vi "QuickSearch Demo.vi"() -> ()   [LabVIEW 2018]
panel:
  in  "Command":string(combo)
  in  "Name Match List":i32(listbox)
  in  "Forward":bool
  in  "Name Match List Ref":refnum<vi>
  in  "Object Name Ref":refnum<vi>
  out "Selected String":string
  out "Shortcuts":string[](array[string])
  in  "vi reference":refnum<vi>
  out "Name":string
  in  "Done":bool
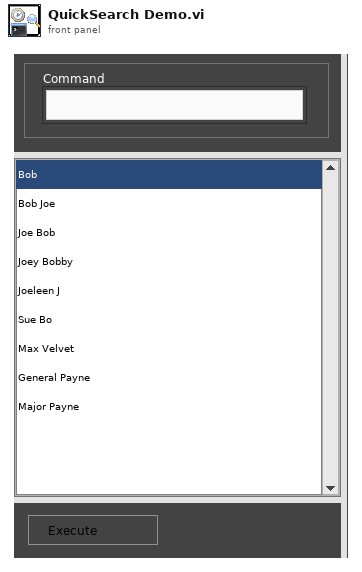
[diagram p1: front panel]
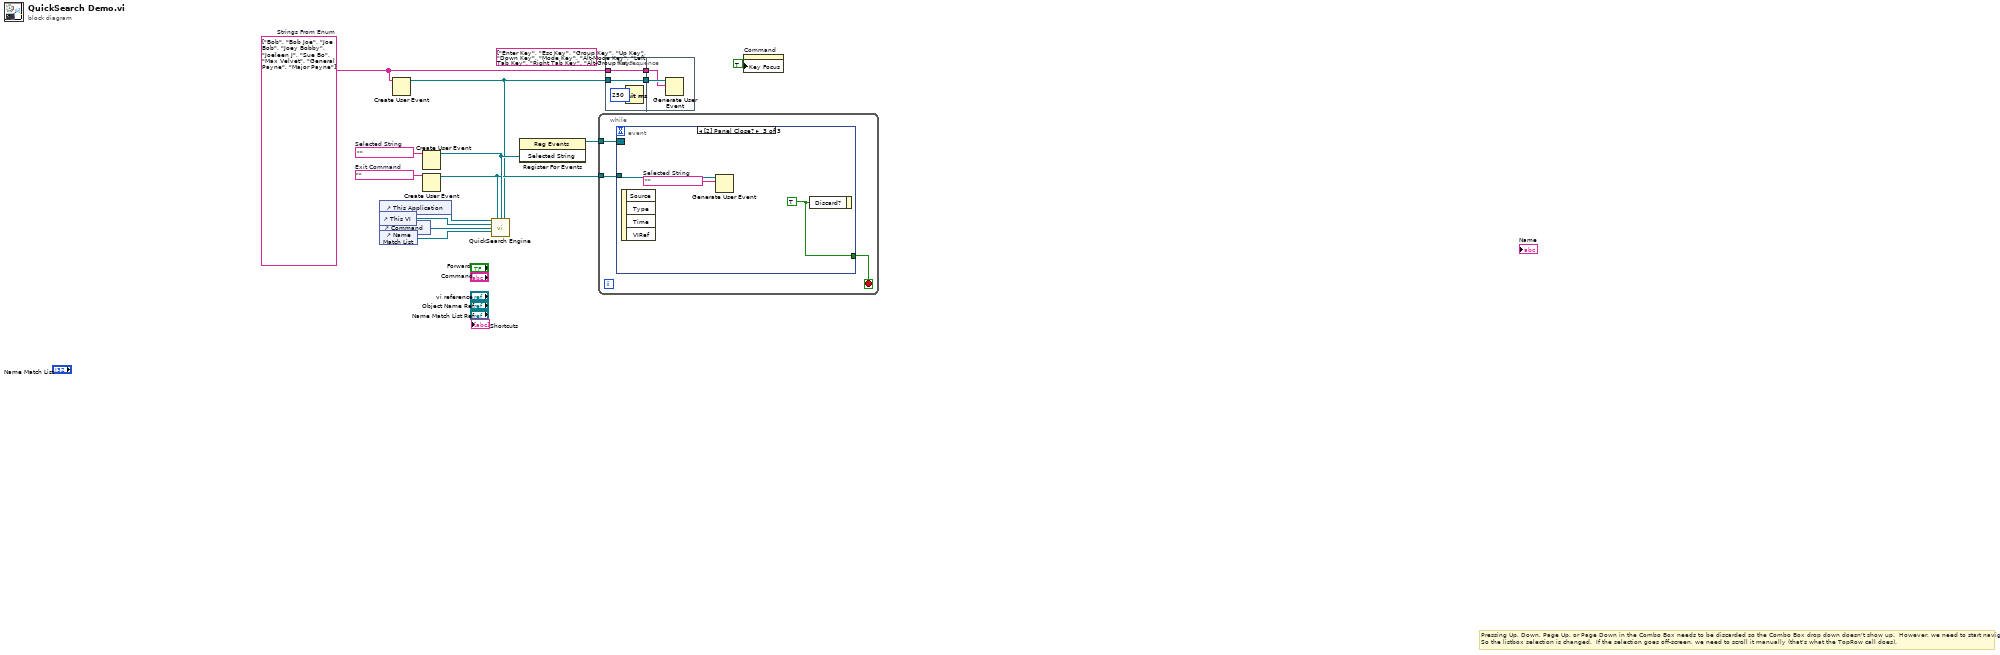
[diagram p0: block diagram]
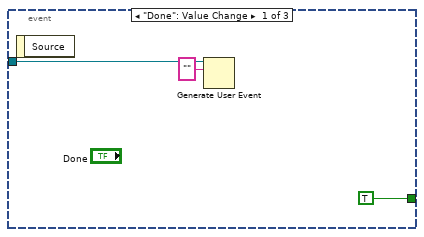
[diagram p2: hidden frame]
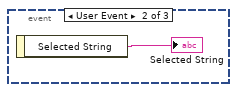
[diagram p3: hidden frame]
diagram:
  w1 = string[] ["Bob", "Bob Joe", "Joe Bob", "Joey Bobby", "Joeleen J", "Sue Bo", "Max Velvet", "General Payne", "Major Payne"]  # Strings From Enum
  (unwired) string[] ["Enter Key", "Esc Key", "Group Key", "Up Key", "Down Key", "Mode Key", "Alt-Mode Key", "Left Tab Key", "Right Tab Key", "Alt-Group Key", "Alt-Enter Key", "Squelch Press", "Squelch Level ", "Programable 1 Key", "Programable 2 Key", "Lock Key", "Set COMSEC", "PTT ON/OFF", "Set Channel Number", "Set Volume", "Set External Port Audio Path", "Set Tone Amplitude", "Set AudioPath-Int/Ext", "Set Traffic Mode (Voice/Data)", "Set Group Number", "Get Supply Voltage", "Get Battery Threshold", "VA Mode - Key Lock Icon", "VA Mode - Channel Knob", "Get Transmit Power", "Set Retransmit Mode", "Get Retransmit Mode", "Get Signal Level", "Set ANDVT Time Delay", "Set VA Mode", "Set WRU Value", "Send Commercial GPS Information", "Set Factory Default Settings", "Set Tx/Rx Frequency", "Set Tx Frequency", "Set Tx Power Level", "Set Tx/Rx CTCSS Tone", "Set Tx CTCSS Tone", "Set Radio Mode", "Get Channel Info", "Set Transmit Timeout", "Set Modulation Type", "Set Traffic Rate", "Set Repeater Delay", "Set Fade Delay", "Set Phase Delay", "Set Squelch Threshold", "Set Beacon Frequency", "Set Beacon ON Time", "Set Beacon OFF Time", "Set Beacon Control_ON_OFF", "Set Hopping Net/Operating Freq(Khz)", "Initialize TOD (HQ Only)", "Set COMSEC Key", "Set Transmit SA", "Set Receive SA", "Set Combat ID", "Set ECCM Mode", "Get ECCM Mode", "Get Software Module Status", "Get Calculated CRC", "Get Elapsed Time", "Reset Elapsed Time", "Set Real Time Clock", "Get Real Time Clock", "Set SINCGARS Net/Channel", "Set SINCGARS Offset", "Set SINCGARS Data Rate", "Get Software Version", "Get Serial Number", "Set Radio To Test Mode", "Software Download Ready Query", "P25 - Get Radio Unit ID", "P25 - Set Transmit NAC", "P25 - Set Receive NAC", "P25 - Set Transmit TGID", "P25 - Set Receive TGID", "P25 - Set Transmit Unit ID", "P25 - Set Squelch Mode", "P25 - Set Operational Mode", "P25 - Set Call Type", "Factory Configuration Query", "Start Continuous Battery Authentication", "Battery Authentication Attempts Query", "P25 - BER Receive Test", "P25 - Transmit Tone Test", "AR - Get Combat ID", "AR - Get Volume", "AR - Set Transmit Power", "AR - Set COMSEC Control", "AR - Get COMSEC Control", "AR - Set COMSEC to TEMP", "AR - Get COMSEC Keyload", "AR - Set CSMA Precedence", "AR - Get CSMA Precedence", "AR - Set CSMA Inter-Transmit Delay", "AR - Get CSMA Inter-Transmit Delay", "AR - Set ICC", "AR - Get ICC", "AR - Set Data Rate", "AR - Get Data Rate", "AR - Set Whisper Mode", "AR - Get Whisper Mode", "AR - Get SC Frequency", "AR - Get SINCGARS Offset", "AR - Set SINCGARS Mode", "AR - Get SINCGARS Mode", "AR - Get SINCGARS Net/Channel", "AR - Set Scan Priority Channel", "AR - Set Scan List", "AR - Set LateNetEntry (LNE)", "AR - Get LateNetEntry (LNE)", "AR - Get COMSEC Key", "AR - Get Freq Hopping Net ID", "LIB - Repeat Last Command", "LIB - Set Channel Operating Mode", "LIB - Set Audio Calibration Value", "LIB - Set RS-232 Baud Rate", "LIB - Reload HW Calibration", "LIB - Feature Display", "LIB - Set LCD Contrast", "LIB - Set LCD Brightness", "LIB - Data Registration Control (OTAR)", "LIB - DTMF Control", "LIB - Emergency Channel Control", "LIB - Set Emergency Channel", "LIB - Set Encryption Functionality", "LIB - Activate Initialized BIT", "LIB - Individual Call Control", "LIB - Set Individual Call Dest. ID", "LIB - Internal Speaker MUTE Control", "LIB - Key Echo Control", "LIB - OTAR Control", "LIB - OTAR Re-key Control", "LIB - Global Talkaround Control", "LIB - Transmit Timeout Control", "My Test", "Set Audio Power", "Initialize port", "Release port"] ("Strings []")
  w2 = ""  # Exit Command
  w3 = ""  # Selected String
  # "Pressing Up, Down, Page Up, or Page Down in the Combo Box needs to be discarded so the Combo Box drop down doesn't show up.  However, we need to start navigating the listbox.  So the listbox selection is changed.  If the selection goes off-screen, we need to scroll it manually (that's what the TopRow call does)."
  n1 = control-ref of="This Application"() -> (w14:refnum<vi>)
  n2 = control-ref of="This VI"() -> (w13:refnum<vi>)
  n3 = control-ref of="Command"() -> (w12:refnum<vi>)
  n4 = control-ref of="Name Match List"() -> (w11:refnum<vi>)
  n5 = Create User Event(user event datatype=w1) -> (user event=w7:refnum<user-event>)  [unwired: 1 in, 1 out]
  n6 = Create User Event(user event datatype=w3) -> (user event=w9:refnum<user-event>)  [unwired: 1 in, 1 out]
  n7 = Create User Event(user event datatype=w2) -> (user event=w8:refnum<user-event>)  [unwired: 1 in, 1 out]
  n8 = call "QuickSearch Engine.vi"("Owning Application"=w14, "Exit Command"=w8, "Selected String"=w9, "New Match List"=w7, "Owning VI"=w13, "Object Name"=w12, "Name Match List"=w11) -> ()  [unwired: 9 in]
  n9 = register-events(w9) -> (reference out=w10:refnum<event-registration>)  [unwired: 2 in, 1 out]
  n10 = while {
    tunnel: w10 -> [w16]
    tunnel: w8 -> [w15]
    stop <- w17 stop-if-true
    n11 = event shown="[2] Panel Close?" {
      selector: w16 -> [_ _ _]
      dyn-events: _ -> [_ _ _]
      timeout: _ -> [_ _ _]
      tunnel: [TRUE _ w24] -> w17
      tunnel: w15 -> [w19 _ w23]
      event "Done": Value Change {
        n12 = event-data() -> ()  [unwired: 1 in, 1 out]
        n13 = Generate User Event(user event=w19, event data cluster="" ("event data")) -> ()  [unwired: 2 in, 2 out]
      }
      event User Event {
        n14 = event-data() -> ("Selected String"=→"Selected String":string)  [unwired: 1 in]
      }
      event Panel Close? {
        w22 = ""  # Selected String
        w24 = TRUE ("Discard?")
        n15 = event-data() -> ()  [unwired: 1 in, 4 out]
        n16 = Generate User Event(user event=w23, event data cluster=w22) -> ()  [unwired: 2 in, 2 out]
        n17 = event-data("Discard?"=w24) -> ()  [unwired: 1 in, 1 out]
      }
    }
  }
  n18 = flat-sequence {
    tunnel: w7 -> [w26]
    tunnel: w1 -> [w27]
    tunnel: [w27] -> w6
    tunnel: [w26] -> w5
    tunnel: w6 -> [w28]
    tunnel: w5 -> [w29]
    frame #0 {
      n19 = Wait (ms)(milliseconds to wait=u32 250) -> ()  [unwired: 1 out]
    }
    frame #1 {
      n20 = Generate User Event(user event=w29, event data cluster=w28) -> ()  [unwired: 2 in, 2 out]
    }
  }
  n21 = property on="Command" class="CmbBox"("Key Focus"=TRUE) -> ()  [unwired: 2 in, 2 out]
